vi "Write active.vi"(8 "error in (no error)":errorcluster, 10 "active":bool, 11 "Component-A in":refnum<class "Component-A.lvclass">) -> (0 "error out":errorcluster, 3 "Component-A out":refnum<class "Component-A.lvclass">)   [LabVIEW 2018, in "Component-A.lvclass"]
uses:
  Component-A.lvclass
  Component-A.lvclass/Component-A.ctl
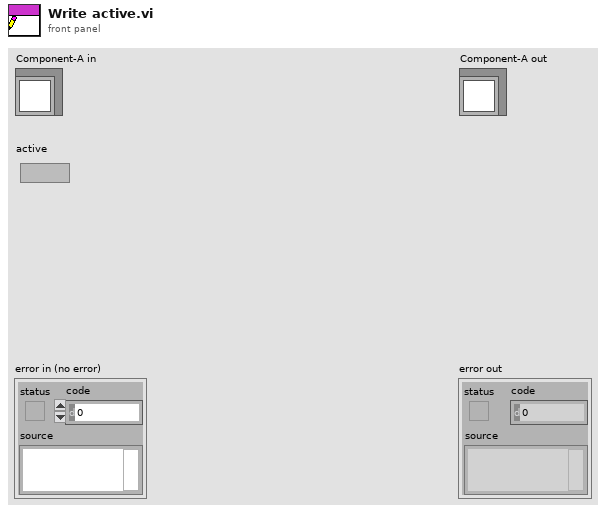
[diagram p1: front panel]
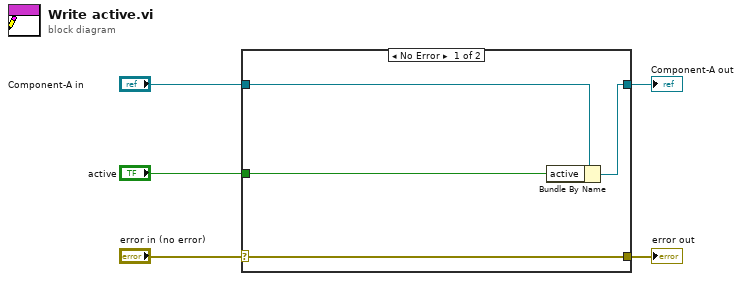
[diagram p0: block diagram]
diagram:
  n1 = case shown="No Error" "error in (no error)" {
    selector: "error in (no error)" -> [w9 w10]
    tunnel: [w9 w10] -> w4
    tunnel: [w7 w11] -> w2
    tunnel: "Component-A in" -> [w8 w11]
    tunnel: "active" -> [w6 _]
    frame No Error {
      n2 = Bundle By Name(cluster=w8, "active"=w6) -> (w7:refnum<class "Component-A.lvclass">)
    }
    frame Error {
    }
  }
  "error out" <- w4
  "Component-A out" <- w2
